vi "Demo_2.vi"() -> ()   [LabVIEW 2020]
uses:
  <vilib>/Waveform/WDTFileIO.llb/Export Waveforms To Spreadsheet File (1D).vi
panel:
  out "data":dynamicdata(graph)
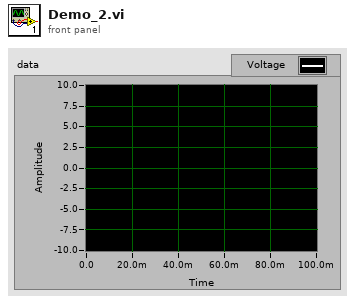
[diagram p1: front panel]
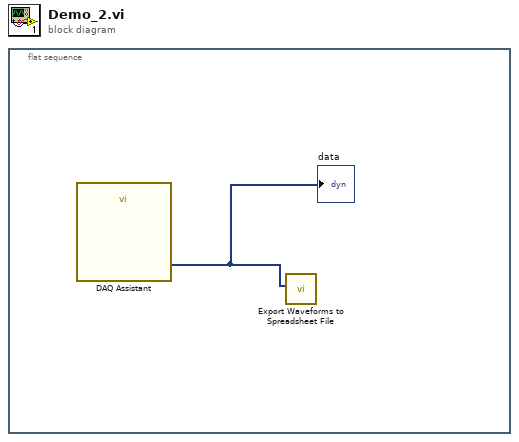
[diagram p0: block diagram]
diagram:
  n1 = flat-sequence {
    frame #0 {
      n2 = call "DAQ Assistant"() -> ("data"=w1:dynamicdata)  [unwired: 17 in, 2 out]
      "data" <- w1
      n3 = call-poly <vilib>:"Export Waveforms to Spreadsheet File.vi"("waveforms"=w1) -> ()  [unwired: 9 in, 2 out]
    }
  }
